vi "GET.comics.series.vi"(7 "timeout (0 = Use Default)":i32=20000, 8 "error in (no error)":errorcluster, 11 "series json path":path) -> (0 "error out":errorcluster, 3 "series json path 2":path)   [LabVIEW 2024]
uses:
  <vilib>/addons/_JKI.lib/REST Client/classes/REST Client/REST Client.lvclass
  <vilib>/addons/_JKI.lib/Serialization/JSON/JKI JSON Serialization.lvlib
panel:
  out "status":string
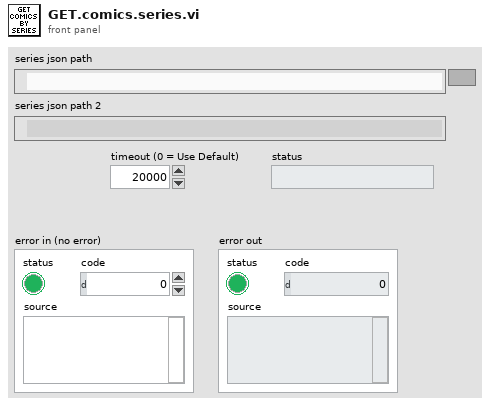
[diagram p1: front panel]
types:
  T1 = enum16{"open", "replace", "create", "open or create", "replace or create", "replace or create with confirmation"}
  T2 = typedef "comics.reply--cluster.ctl" = cluster{"code":i32, "status":string, "etag":string, "data":cluster{"offset":i32, "limit":i32, "total":i32, "count":i32, "results":T3[]}}
  T3 = typedef "comic--cluster.ctl" = cluster{"id":i32, "digitalId":i32, "title":string, "issueNumber":i32, "variantDescription":string, "description":string, "modified":variant, "upc":string, "format":string, "pageCount":i32, "resourceURI":string, "urls":cluster{"type":string, "url":string}[], "series":cluster{"resourceURI":string, "name":string}, "dates":cluster{"type":string, "date":string}[], "prices":cluster{"price":dbl, "type":string}[], "thumbnail":cluster{"path":string, "extension":string}, "images":cluster{"path":string, "extension":string}[], "creators":cluster{"available":i32, "returned":i32, "collectionURI":string, "items":cluster{"resourceURI":string, "name":string, "role":string}[]}, "characters":cluster{"available":i32, "returned":i32, "collectionURI":string, "items":cluster{"resourceURI":string, "name":string}[]}, "stories":cluster{"available":i32, "returned":i32, "collectionURI":string, "items":cluster{"resourceURI":string, "name":string, "type":string}[]}, "events":cluster{"available":i32, "returned":i32, "collectionURI":string, "items":cluster{"resourceURI":string, "name":string}[]}}
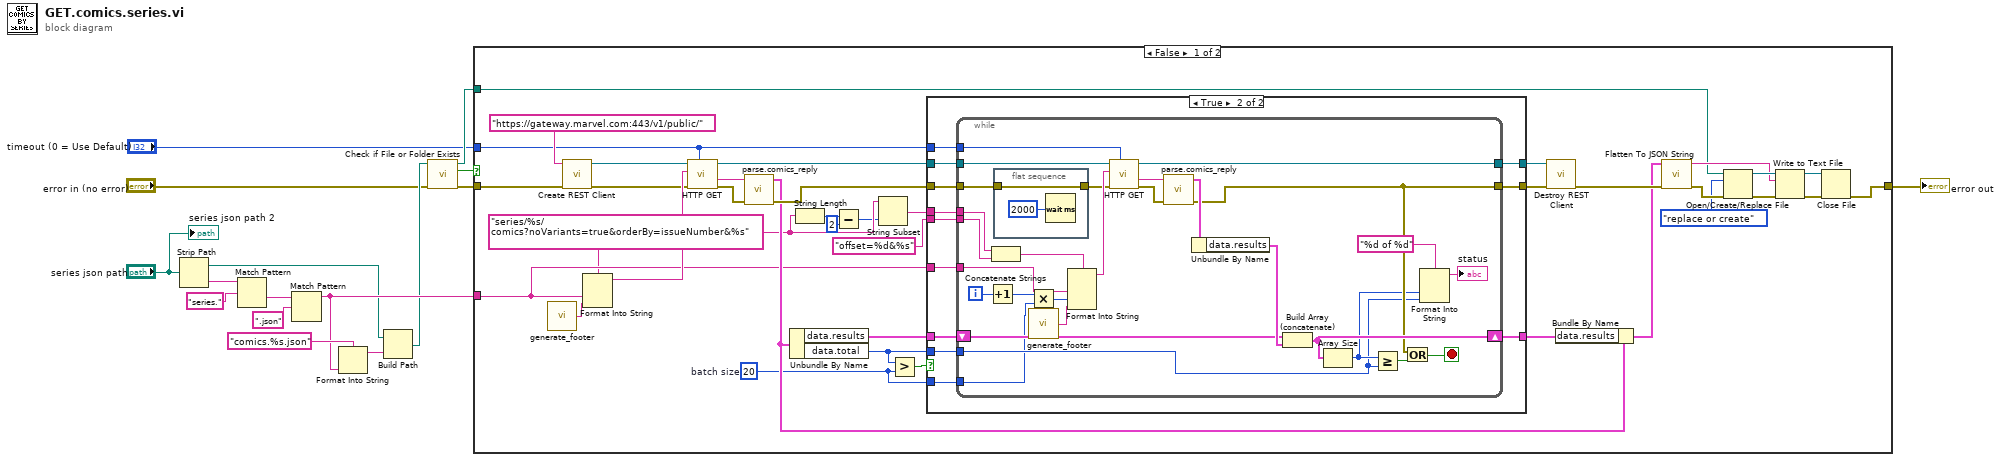
[diagram p0: block diagram]
diagram:
  n1 = Strip Path(path="series json path") -> (stripped path=w7:path, name=w15:string)
  n2 = Match Pattern(string=w15, regular expression="series.") -> (after substring=w13:string)  [unwired: 1 in, 3 out]
  n3 = Match Pattern(string=w13, regular expression=".json") -> (before substring=w9:string)  [unwired: 1 in, 3 out]
  n4 = Format Into String(format string="comics.%s.json", w9) -> (resulting string=w8:string)  [unwired: 2 in, 1 out]
  n5 = Build Path(base path=w7, name or relative path=w8) -> (appended path=w6:path)
  n6 = call <vilib>:"Check if File or Folder Exists.vi"("error in (no error)"="error in (no error)", "path"=w6) -> ("error out"=w4:errorcluster, "file or folder exists?"=w2:bool, "dup path"=w3:path)  [unwired: 7 in]
  n7 = case shown="False" w2 {
    tunnel: [w27 w99] -> w11
    tunnel: w9 -> [w24 _]
    tunnel: w4 -> [w26 w99]
    tunnel: w3 -> [w25 _]
    tunnel: "timeout (0 = Use Default)" -> [w18 _]
    frame False {
      w17 = 20  # batch size
      w23 = "series/%s/comics?noVariants=true&orderBy=issueNumber&%s" ("Path")
      n8 = call "generate_footer.vi"() -> ("footer"=w47:string)  [unwired: 1 in]
      n9 = call <vilib>:"Create REST Client.vi"("error in (no error)"=w26, "Base URL"="https://gateway.marvel.com:443/v1/public/") -> ("error out"=w48:errorcluster, "REST Client out"=w49:refnum<class "REST Client.lvclass">)  [unwired: 8 in]
      n10 = Format Into String(format string=w23, w24, w47) -> (resulting string=w51:string)  [unwired: 2 in, 1 out]
      n11 = call-dynamic "HTTP GET.vi"("timeout (0 = Use Default)"=w18, "error in (no error)"=w48, "Path"=w51, "REST Client in"=w49) -> ("error out"=w53:errorcluster, "Response body"=w52:string, "REST Client out"=w45:refnum<class "REST Client.lvclass">)  [unwired: 2 in, 3 out]
      n12 = call "parse.comics_reply.vi"("error in"=w53, "string in"=w52) -> ("error out"=w43:errorcluster, "data"=w40:T2)  [unwired: 8 in]
      n13 = Unbundle By Name(w40) -> ("data.results"=w41:T3[], "data.total"=w37:i32)
      n14 = String Length(string=w23) -> (length=w21:i32)
      n15 = Subtract(x=w21, y=2) -> (x-y=w19:i32)
      n16 = String Subset(string=w23, length (rest)=w19) -> (substring=w22:string)  [unwired: 1 in]
      n17 = Greater?(x=w37, y=w17) -> (0:w46:bool)
      n18 = case shown="True" w46 {
        tunnel: [w56 w63] -> w44
        tunnel: w45 -> [w56 w66]
        tunnel: [w55 w61] -> w42
        tunnel: w43 -> [w55 w62]
        tunnel: w41 -> [w54 w68]
        tunnel: [w54 w67] -> w39
        tunnel: w22 -> [_ w65]
        tunnel: "offset=%d&%s" -> [_ w64]
        tunnel: w37 -> [_ w60]
        tunnel: w24 -> [_ w59]
        tunnel: w18 -> [_ w58]
        tunnel: w17 -> [_ w57]
        frame False {
        }
        frame True {
          n19 = while {
            shift-right: [w82] -> w67
            shift-left: w68 -> [w83]
            tunnel: w66 -> [w90]
            tunnel: w65 -> [w95]
            tunnel: w64 -> [w96]
            tunnel: [w89] -> w63
            tunnel: w62 -> [w70]
            tunnel: [w80] -> w61
            tunnel: w60 -> [w75]
            tunnel: w59 -> [w78]
            tunnel: w58 -> [w73]
            tunnel: w57 -> [w72]
            i -> [w92]
            stop <- w79 stop-if-true
            n20 = Increment(x=w92) -> (x+1=w71:i32)
            n21 = Concatenate Strings(w95, w96) -> (w94:string)
            n22 = flat-sequence {
              tunnel: w70 -> [w98]
              tunnel: [w98] -> w69
              frame #0 {
                n23 = Wait (ms)(milliseconds to wait=u32 2000) -> ()  [unwired: 1 out]
              }
            }
            n24 = Multiply(x=w71, y=w72) -> (x*y=w91:i32)
            n25 = call "generate_footer.vi"() -> ("footer"=w93:string)  [unwired: 1 in]
            n26 = Format Into String(format string=w94, w78, w91, w93) -> (resulting string=w86:string)  [unwired: 2 in, 1 out]
            n27 = call-dynamic "HTTP GET.vi"("timeout (0 = Use Default)"=w73, "error in (no error)"=w69, "Path"=w86, "REST Client in"=w90) -> ("error out"=w87:errorcluster, "Response body"=w88:string, "REST Client out"=w89:refnum<class "REST Client.lvclass">)  [unwired: 2 in, 3 out]
            n28 = call "parse.comics_reply.vi"("error in"=w87, "string in"=w88) -> ("error out"=w80:errorcluster, "data"=w85:T2)  [unwired: 8 in]
            n29 = Unbundle By Name(w85) -> ("data.results"=w84:T3[])
            n30 = Build Array (concatenate)(w83, w84) -> (w82:T3[])
            n31 = Array Size(array=w82) -> (size(s)=w76:i32)
            n32 = Greater Or Equal?(x=w76, y=w75) -> (x >= y?=w81:bool)
            n33 = Or(x=w80, y=w81) -> (x .or. y?=w79:bool)
            n34 = Format Into String(format string="%d of %d", w76, w75) -> (resulting string=→"status":string)  [unwired: 2 in, 1 out]
          }
        }
      }
      n35 = call-dynamic "Destroy REST Client.vi"("error in (no error)"=w42, "REST Client in"=w44) -> ("error out"=w36:errorcluster)  [unwired: 9 in]
      n36 = Bundle By Name(cluster=w40, "data.results"=w39) -> (w35:T2)
      n37 = call <vilib>:"Flatten To JSON String.vi"("error in (no error)"=w36, "Variant"=w35) -> ("error out"=w34:errorcluster, "JSON String"=w30:string)  [unwired: 8 in]
      n38 = Open/Create/Replace File(file path (use dialog)=w25, error in=w34, operation (0:open)=T1."replace or create") -> (refnum out=w31:refnum<file>, error out=w32:errorcluster)  [unwired: 3 in, 1 out]
      n39 = Write to Text File(file (use dialog)=w31, text=w30, error in=w32) -> (refnum out=w28:refnum<file>, error out=w29:errorcluster)  [unwired: 1 in, 1 out]
      n40 = Close File(refnum=w28, error in=w29) -> (error out=w27:errorcluster)  [unwired: 1 out]
    }
    frame True {
    }
  }
  "error out" <- w11
  "series json path 2" <- "series json path"
